vi "Do.vi"(8 "error in (no error)":errorcluster, 10 "Actor in":refnum<class "Actor.lvclass">, 11 "UI Front Panel State Msg":refnum<class "UI Front Panel State Msg.lvclass">) -> (0 "error out":errorcluster, 2 "Actor out":refnum<class "Actor.lvclass">)   [LabVIEW 2021, in "AbstractActorTemplate.lvlib" / "UI Front Panel State Msg.lvclass"]
doc: "This VI delivers the message to the actor by calling the appropriate method(s) on the actor."
uses:
  <userlib>/John_Lib/AbstractActorTemplate/UIActorTop Messages/UI Front Panel State Msg/UI Front Panel State Msg.lvclass
  <userlib>/John_Lib/AbstractActorTemplate/UIActorTop Messages/UI Front Panel State Msg/UI Front Panel State Msg.lvclass/UI Front Panel State Msg.ctl
  9ef47adc-f318-494c-9b8b-6df3216d6863.vi
  <userlib>/John_Lib/AbstractActorTemplate/AbstractActorTemplate/UIActorTop.lvclass
  <vilib>/ActorFramework/Actor/Actor.lvclass
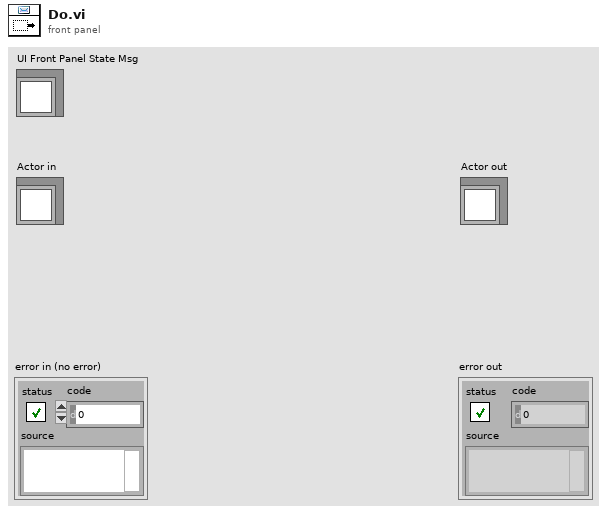
[diagram p1: front panel]
types:
  T1 = typedef "sushu.lvlib/Front Panel State.ctl" = string
  T2 = enum32{"Invalid", "Default", "Floating", "Floating/Auto-Hide", "Modal"}
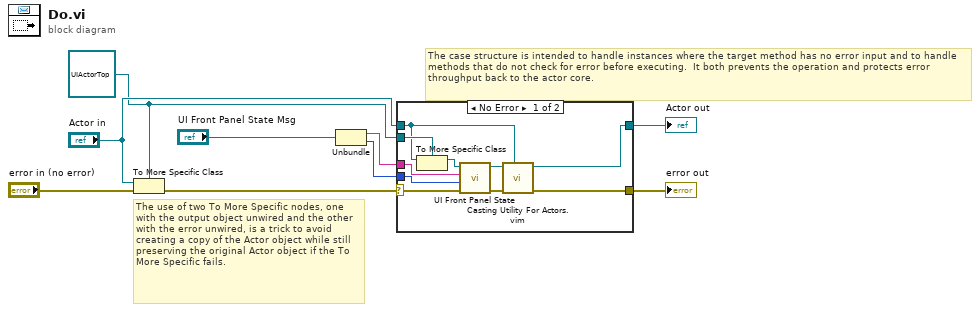
[diagram p0: block diagram]
diagram:
  w3 = refnum<class "UIActorTop.lvclass"> refnum ("Actor in")
  # "The use of two To More Specific nodes, one with the output object unwired and the other with the error unwired, is a trick to avoid creating a copy of the Actor object while still preserving the original Actor object if the To More Specific fails."
  # "The case structure is intended to handle instances where the target method has no error input and to handle methods that do not check for error before executing.  It both prevents the operation and protects error throughput back to the actor core."
  n1 = To More Specific Class(target class=w3, reference="Actor in", error in="error in (no error)") -> (error out=w7:errorcluster)  [unwired: 1 out]
  n2 = Unbundle("UI Front Panel State Msg") -> (w2:T1, w1:T2)
  n3 = case shown="No Error" w7 {
    selector: w7 -> [w19 w21]
    tunnel: [w13 w21] -> w6
    tunnel: [w14 w20] -> w5
    tunnel: "Actor in" -> [w16 w20]
    tunnel: w3 -> [w17 _]
    tunnel: w2 -> [w11 _]
    tunnel: w1 -> [w10 _]
    frame No Error {
      n4 = To More Specific Class(target class=w17, reference=w16) -> (specific class reference=w18:refnum<class "UIActorTop.lvclass">)  [unwired: 1 in, 1 out]
      n5 = call-dynamic "UI Front Panel State.vi"("error in (no error)"=w19, "Front Panel Window:Behavior"=w10, "Argument"=w11, "UI ActorTop in"=w18) -> ("error out"=w12:errorcluster, "UI ActorTop out"=w15:refnum<class "UIActorTop.lvclass">)  [unwired: 6 in]
      n6 = call "Casting Utility For Actors.vim"("type"=w16, "error in (no error)"=w12, "Actor in"=w15) -> ("error out"=w13:errorcluster, "Actor out"=w14:refnum<class "Actor.lvclass">)  [unwired: 7 in]
    }
    frame Error {
      # "If type check fails, pass the original object out again."
    }
  }
  "error out" <- w6
  "Actor out" <- w5
